vi "Msg To.vi"(10 "Error":errorcluster) -> (3 "Merge Error Msg Strategy out":refnum<class "Merge Error Msg Strategy.lvclass">)   [LabVIEW 2021, in "jettl.lvlib" / "Merge Error.lvlib"]
uses:
  Merge Error.lvlib
  Merge Error Msg Strategy/Merge Error Msg Strategy.lvclass
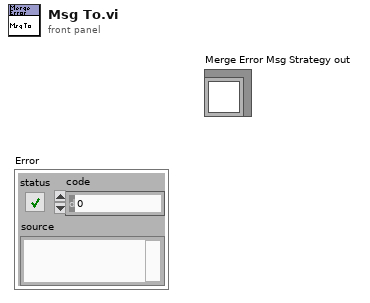
[diagram p1: front panel]
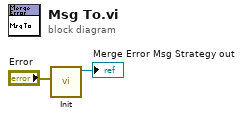
[diagram p0: block diagram]
diagram:
  n1 = call "Init.vi"("Error"="Error") -> ("Merge Error Msg Strategy out"=→"Merge Error Msg Strategy out":refnum<class "Merge Error Msg Strategy.lvclass">)  [unwired: 10 in]
